vi "Process data magnetometer.vi"() -> ()   [LabVIEW 2021]
uses:
  <vilib>/Platform/TimedLoop/XDataNode/timing_clust.ctl
  <vilib>/Platform/TimedLoop/XDataNode/nitl_modes.ctl
  <vilib>/Platform/TimedLoop/XDataNode/wakeup.ctl
  <vilib>/picture/3D Picture Control/Object/Create Object (name).vi
  <vilib>/picture/3D Picture Control/Object/Create Object (drawable).vi
  <vilib>/picture/3D Picture Control/Object/Add Object (no reference).vi
  <vilib>/platform/TimedLoop/XDataNode/XDataNode.xnode
  <vilib>/Platform/TimedLoop/XDataNode/XDNodeRunTimeDep.lvlib
  <vilib>/gmath/NI_Gmath.lvlib
  <vilib>/picture/3D Picture Control/NI_3D Picture Control.lvlib
panel:
  out "Numeric":i32
  in  "Clear":bool
  in  "Calibrate":bool
  out "Magnetometer corrected":refnum<vi>(3d-picture)
  out "Magnetometer":refnum<vi>(3d-picture)
  in  "stop":bool
  in  "DAQ Port":refnum<visa-resource-name>
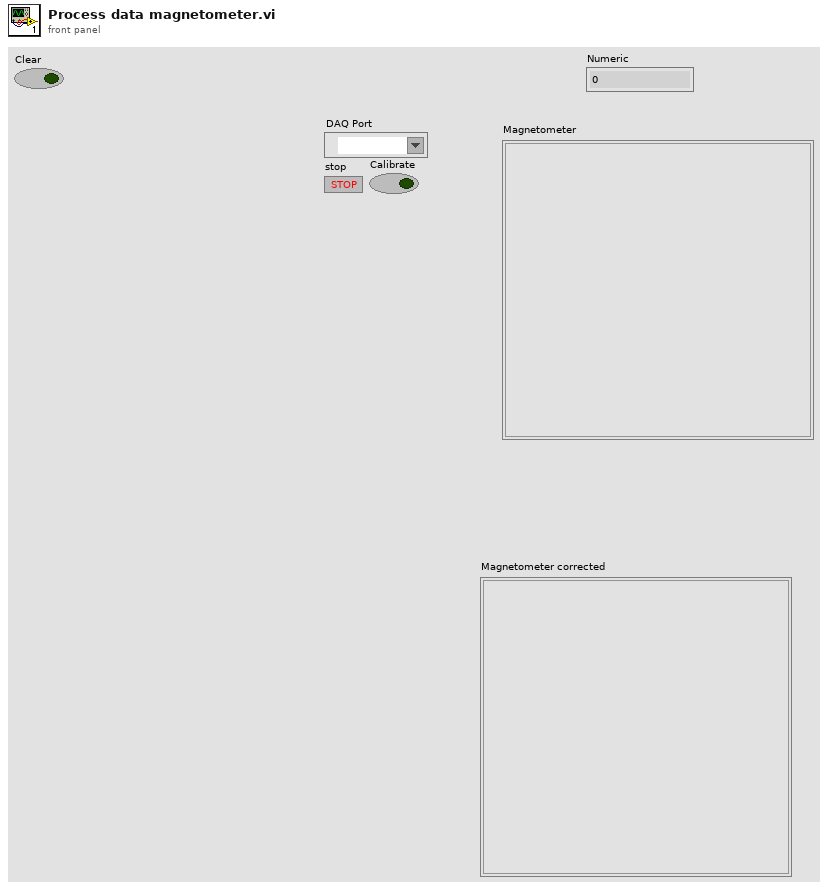
[diagram p1: front panel]
types:
  T1 = cluster{"Red":sgl, "Green":sgl, "Blue":sgl, "Alpha":sgl}
  T2 = typedef "XDNodeRunTimeDep.lvlib/timing_clust.ctl" = cluster{"Expected End [f-1]":u64, "Actual End [f-1]":u64, "Finished Late? [f-1]":bool, "Expected End [i-1]":u64, "Actual End [i-1]":u64, "Finished Late? [i-1]":bool, "Expected Start [i]":u64, "Actual Start [i]":u64, "Expected Start [f]":u64, "Actual Start [f]":u64, "Source Name":string, "Structure Name":string, "Period":i64, "Deadline":i64, "Offset":i64, "Start":i64, "Priority":i32, "Timeout":i32, "Mode":T3, "Wakeup Reason":T4, "Error":errorcluster, "Source Type":string, "Secondary Source Type":string, "Global End Time":u64, "Global Start Time":u64, "Frame Duration":u64, "Iteration Duration":u64, "Assigned CPU":i32, "I/O Scan Engine Mode":u32}
  T3 = typedef "XDNodeRunTimeDep.lvlib/nitl_modes.ctl" = enum32{"No Change", "Process missed periods, maintain original phase", "Discard missed periods, maintain original phase", "Process missed periods, ignore original phase", "Discard missed periods, ignore original phase"}
  T4 = typedef "XDNodeRunTimeDep.lvlib/wakeup.ctl" = enum32{"Normal", "Aborted", "Asynchronous wakeup", "Timing source error", "Timed loop error", "Timeout"}
  T5 = cluster{"x0, y0, z0[0]":dbl, "x0, y0, z0[1]":dbl, "x0, y0, z0[2]":dbl}
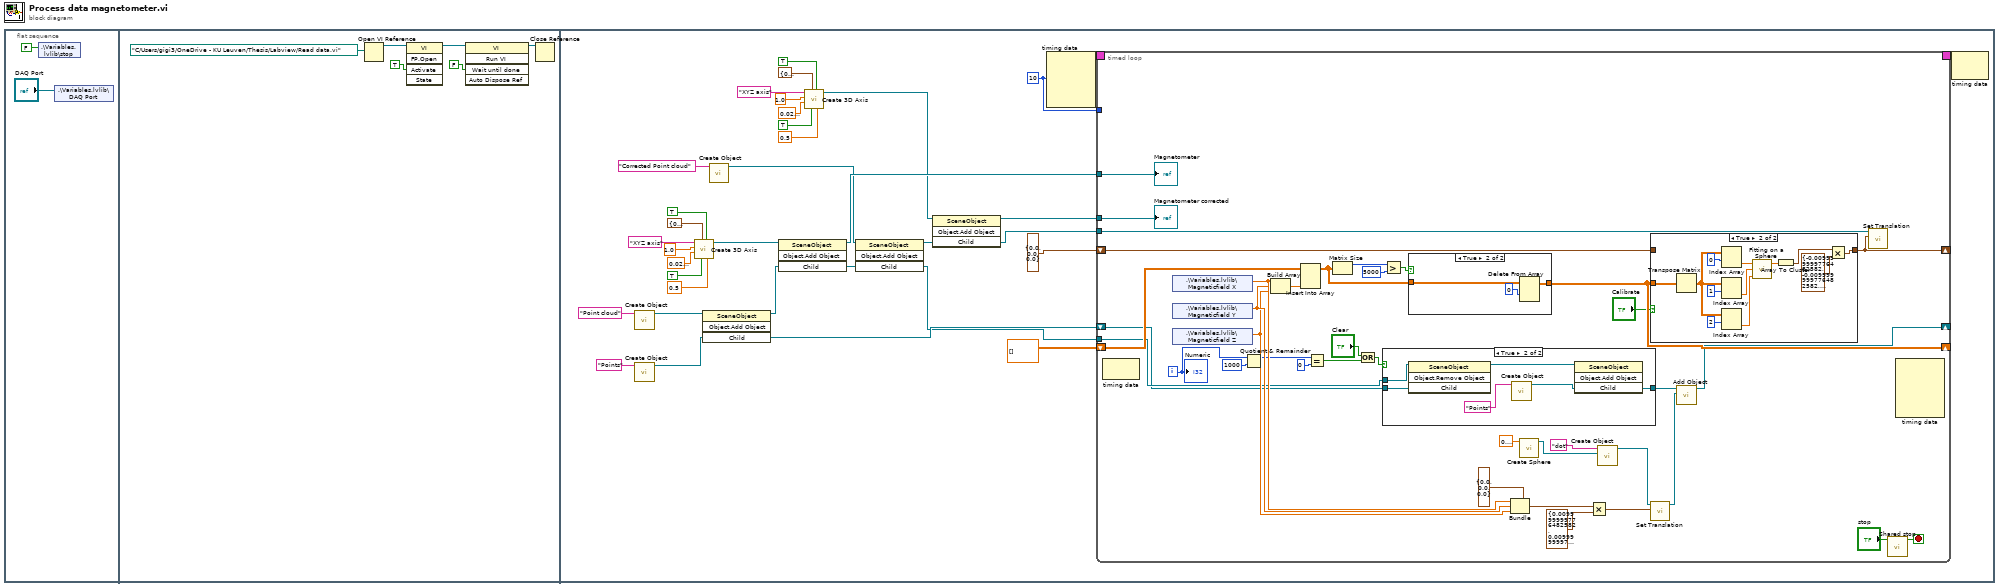
[diagram p0: block diagram]
diagram:
  n1 = flat-sequence {
    frame #0 {
      n2 = shared-variable ".\\Variables.lvlib\\stop"(FALSE ("stop")) -> ()  [unwired: 1 in, 1 out]
      n3 = shared-variable ".\\Variables.lvlib\\DAQ Port"("DAQ Port") -> ()  [unwired: 1 in, 1 out]
    }
    frame #1 {
      n4 = Open VI Reference(vi path=path "C:/Users/gigi3/OneDrive - KU Leuven/Thesis/Labview/Read data.vi") -> (vi reference=w8:refnum<vi>)  [unwired: 5 in, 1 out]
      n5 = invoke class="VI" method="FP.Open"(reference=w8, "Activate"=TRUE ("Activate?")) -> (reference out=w7:refnum<vi>)  [unwired: 3 in, 4 out]
      n6 = invoke class="VI" method="Run VI"(reference=w7, "Wait until done"=FALSE ("Wait Until Done")) -> (reference out=w4:refnum<vi>)  [unwired: 3 in, 4 out]
      n7 = Close Reference(reference=w4) -> ()  [unwired: 1 in, 1 out]
    }
    frame #2 {
      w41 = i64 10 ("Period")
      n8 = call-poly <vilib>:"Create Object.vi"("Name"="Point cloud") -> ("Scene:New Object"=w11:refnum<vi>)  [unwired: 9 in, 1 out]
      n9 = call-poly <vilib>:"Create Object.vi"("Name"="Points") -> ("Scene:New Object"=w13:refnum<vi>)  [unwired: 9 in, 1 out]
      n10 = call <vilib>:"Create 3D Axis.vi"("Character Size"=sgl 0.5, "Half plane?"=TRUE, "Axis label?"=TRUE, "Color"=T1 {"Red"=0.0, "Green"=1.0, "Blue"=0.0, "Alpha"=1.0}, "Radius"=sgl 0.03, "Length"=sgl 1.0, "Name"="XYZ axis") -> ("New Object Refnum"=w25:refnum<vi>)  [unwired: 3 in, 1 out]
      n11 = invoke class="SceneObject" method="Object.Add Object"(reference=w11, "Child"=w13) -> (reference out=w12:refnum<vi>, "Child"=w10:refnum<vi>)  [unwired: 2 in, 2 out]
      n12 = call-poly <vilib>:"Create Object.vi"("Name"="Corrected Point cloud") -> ("Scene:New Object"=w21:refnum<vi>)  [unwired: 9 in, 1 out]
      n13 = invoke class="SceneObject" method="Object.Add Object"(reference=w25, "Child"=w12) -> (reference out=w24:refnum<vi>, "Child"=w16:refnum<vi>)  [unwired: 2 in, 2 out]
      n14 = call <vilib>:"Create 3D Axis.vi"("Character Size"=sgl 0.5, "Half plane?"=TRUE, "Axis label?"=TRUE, "Color"=T1 {"Red"=0.0, "Green"=1.0, "Blue"=0.0, "Alpha"=1.0}, "Radius"=sgl 0.03, "Length"=sgl 1.0, "Name"="XYZ axis") -> ("New Object Refnum"=w20:refnum<vi>)  [unwired: 3 in, 1 out]
      n15 = invoke class="SceneObject" method="Object.Add Object"(reference=w21, "Child"=w16) -> (reference out=w19:refnum<vi>, "Child"=w9:refnum<vi>)  [unwired: 2 in, 2 out]
      n16 = invoke class="SceneObject" method="Object.Add Object"(reference=w20, "Child"=w19) -> (reference out=w18:refnum<vi>, "Child"=w17:refnum<vi>)  [unwired: 2 in, 2 out]
      n17 = node-c288(w41) -> (w43:T2)  [unwired: 3 in]
      n18 = timed-loop {
        timing: w43 -> [_]
        timing-out: [_] -> w42
        tunnel: w41 -> [_]
        shift-right: [w75] -> _
        shift-left: dbl[][] [] -> [w80]
        tunnel: w24 -> [w61]
        tunnel: w18 -> [w60]
        tunnel: w17 -> [w59]
        shift-right: [w57] -> _
        shift-left: cluster{dbl, dbl, dbl} {0.0, 0.0, 0.0} -> [w56]
        tunnel: w9 -> [w54]
        shift-right: [w52] -> _
        shift-left: w10 -> [w51]
        i -> [w48]
        stop <- w44 stop-if-true
        n19 = node-c288() -> ()  [unwired: 1 in, 1 out]
        n20 = shared-variable ".\\Variables.lvlib\\Magneticfield X"() -> (w66:dbl)  [unwired: 1 in, 1 out]
        n21 = shared-variable ".\\Variables.lvlib\\Magneticfield Y"() -> (w65:dbl)  [unwired: 1 in, 1 out]
        n22 = shared-variable ".\\Variables.lvlib\\Magneticfield Z"() -> (w64:dbl)  [unwired: 1 in, 1 out]
        n23 = Quotient & Remainder(x=w48, y=1000) -> (x-y*floor(x/y)=w45:i32)  [unwired: 1 out]
        n24 = Build Array(w66, w65, w64) -> (w62:dbl[])
        n25 = Insert Into Array(array=w80, new element=w62) -> (w79:dbl[][])  [unwired: 2 in]
        n26 = Equal?(x=w45, y=0) -> (x = y?=w47:bool)
        n27 = Matrix Size(0:w79) -> (1:w78:i32)  [unwired: 1 out]
        n28 = Or(x="Clear", y=w47) -> (x .or. y?=w50:bool)
        n29 = case shown="True" w50 {
          tunnel: w54 -> [_ w88]
          tunnel: [w82 w83] -> w53
          tunnel: w51 -> [w82 w84]
          frame False {
          }
          frame True {
            n30 = invoke class="SceneObject" method="Object.Remove Object"(reference=w88, "Child"=w84) -> (reference out=w86:refnum<vi>)  [unwired: 2 in, 3 out]
            n31 = call-poly <vilib>:"Create Object.vi"("Name"="Points") -> ("Scene:New Object"=w85:refnum<vi>)  [unwired: 9 in, 1 out]
            n32 = invoke class="SceneObject" method="Object.Add Object"(reference=w86, "Child"=w85) -> ("Child"=w83:refnum<vi>)  [unwired: 2 in, 3 out]
          }
        }
        n33 = Greater?(x=w78, y=5000) -> (0:w76:bool)
        n34 = case shown="True" w76 {
          tunnel: w79 -> [w102 w105]
          tunnel: [w102 w103] -> w75
          frame False {
          }
          frame True {
            n35 = Delete From Array(array=w105, index (row)=0) -> (array with subset deleted=w103:dbl[][])  [unwired: 2 in, 1 out]
          }
        }
        n36 = Bundle(cluster=cluster{"X":sgl, "Y":sgl, "Z":sgl} {"X"=0.0, "Y"=0.0, "Z"=0.0} ("Translation"), "X"=w66, "Y"=w65, "Z"=w64) -> (w69:cluster{"X":sgl, "Y":sgl, "Z":sgl})
        n37 = call <vilib>:"Create Sphere.vi"("Radius"=sgl 0.1) -> ("New Sphere Refnum"=w73:refnum<vi>)  [unwired: 9 in, 1 out]
        n38 = Multiply(x=w69, y=cluster{"X":sgl, "Y":sgl, "Z":sgl} {"X"=0.01, "Y"=0.01, "Z"=0.01}) -> (x*y=w67:cluster{"X":sgl, "Y":sgl, "Z":sgl})
        n39 = call-poly <vilib>:"Create Object.vi"("Geometry"=w73, "Name"="dot") -> ("Scene:New Object"=w71:refnum<vi>)  [unwired: 8 in, 1 out]
        n40 = case shown="True" "Calibrate" {
          tunnel: w75 -> [_ w101]
          tunnel: [w89 w91] -> w57
          tunnel: w56 -> [w89 _]
          frame False {
          }
          frame True {
            n41 = Transpose Matrix(1:w101) -> (0:w96:dbl[][])
            n42 = Index Array(array=w96, index (row)=0) -> (element=w100:dbl[])  [unwired: 1 in]
            n43 = Index Array(array=w96, index (row)=1) -> (element=w95:dbl[])  [unwired: 1 in]
            n44 = Index Array(array=w96, index (row)=2) -> (element=w94:dbl[])  [unwired: 1 in]
            n45 = call <vilib>:"Fitting on a Sphere.vi"("Z"=w94, "Y"=w95, "X"=w100) -> ("x0, y0, z0"=w93:dbl[])  [unwired: 2 out]
            n46 = Array To Cluster(array=w93) -> (cluster=w92:T5)
            n47 = Multiply(x=w92, y=cluster{"X":sgl, "Y":sgl, "Z":sgl} {"X"=-0.01, "Y"=-0.01, "Z"=-0.01}) -> (x*y=w91:cluster{dbl, dbl, dbl})
          }
        }
        n48 = call <vilib>:"Set Translation.vi"("Translation"=w67, "Scene Object"=w71) -> ("Translated Object"=w70:refnum<vi>)  [unwired: 8 in, 1 out]
        n49 = call-poly <vilib>:"Add Object.vi"("New Object In"=w70, "Scene Object In"=w53) -> ("Scene Object Out"=w52:refnum<vi>)  [unwired: 8 in, 1 out]
        n50 = call <vilib>:"Set Translation.vi"("Translation"=w57, "Scene Object"=w59) -> ()  [unwired: 8 in, 2 out]
        n51 = call "Shared stop.vi"("stop"="stop") -> ("stop 2"=w44:bool)  [unwired: 10 in]
        n52 = node-c288() -> ()  [unwired: 5 in, 1 out]
        "Magnetometer" <- w61
        "Magnetometer corrected" <- w60
        "Numeric" <- w48
      }
      n53 = node-c288(w42) -> ()  [unwired: 1 out]
    }
  }
